vi "SLSC Convert EDS Properties and Commands to Tree Control.vi"(4 "Enum string":cluster{"name":string, "enum":string}[](array[cluster]), 6 "Item Indent":i32, 9 "commands":T1[](array[typedef]), 10 "properties":T2[](array[typedef]), 11 "Child Tag":string) -> (3 "Tree Items":T3(array[cluster]))   [LabVIEW 2017, in "SLSC Tree Control.lvlib"]
doc: "Convert the properties and commands datatypes to a Tree Control items."
uses:
  SLSC Tree Control.lvlib
  Ctrl/Property.ctl
  Ctrl/command.ctl
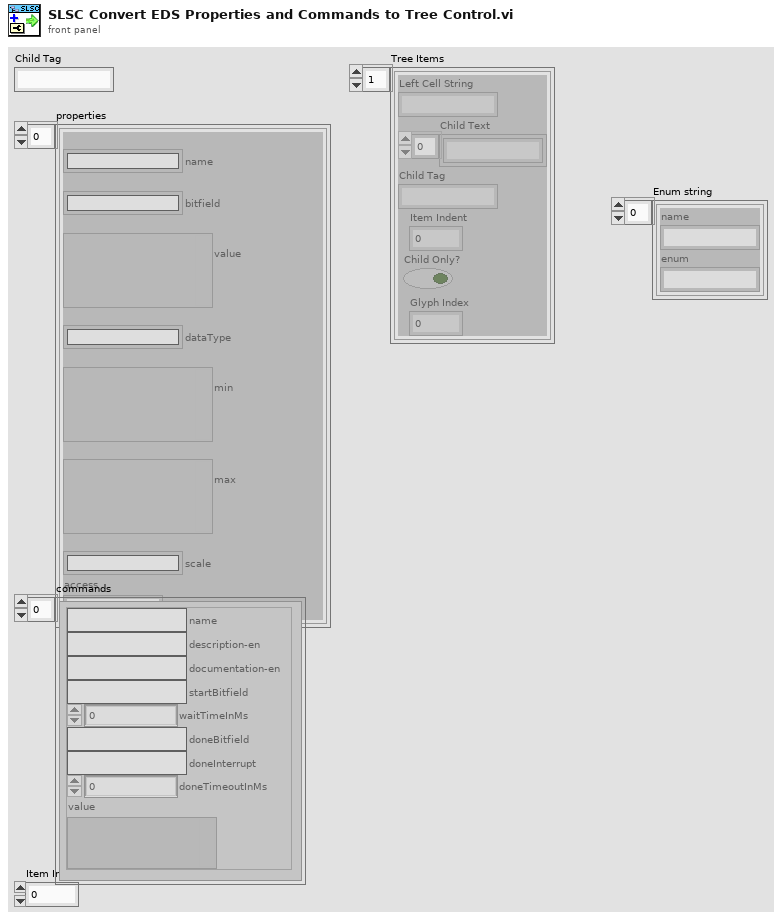
[diagram p1: front panel]
types:
  T1 = typedef "command.ctl" = cluster{"name":string, "description-en":string, "documentation-en":string, "startBitfield":string, "waitTimeInMs":i32, "doneBitfield":string, "doneInterrupt":string, "doneTimeoutInMs":i32, "value":variant}
  T2 = typedef "Property.ctl" = cluster{"name":string, "bitfield":string, "value":variant, "dataType":string, "min":variant, "max":variant, "scale":string, "access":string}
  T3 = cluster{"Left Cell String":string, "Child Text":string[], "Child Tag":string, "Item Indent":i32, "Child Only?":bool, "Glyph Index":i32}[]
  T4 = cluster{"Left Cell String":string, "Child Text":string[], "Child Tag":string, "Item Indent":i32, "Child Only?":bool, "Glyph Index":i32, "offline value":variant}
  T5 = cluster{"Left Cell String":string, "Child Text":string[], "Child Tag":string, "Item Indent":i32, "Child Only?":bool, "Glyph Index":i32, "offline value":variant}[]
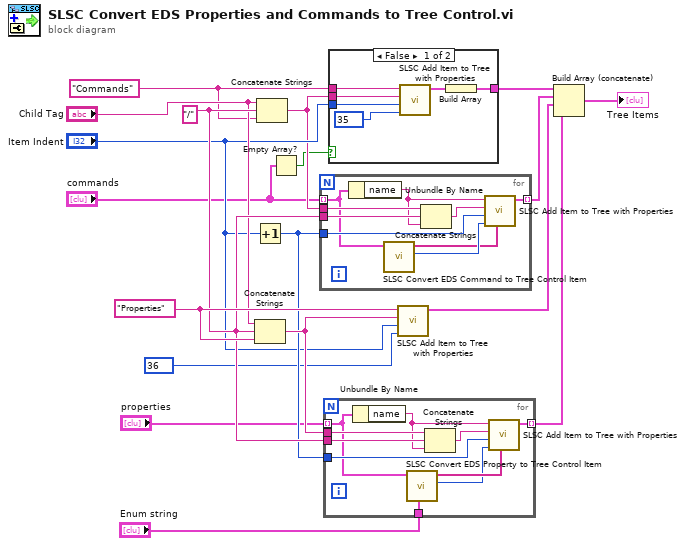
[diagram p0: block diagram]
diagram:
  w16 = "Properties" ("Left Cell String")
  w4 = "Commands" ("Left Cell String")
  w15 = "/" ("string")
  n1 = Increment(x="Item Indent") -> (x+1=w12:i32)
  n2 = Concatenate Strings("Child Tag", w15, w16) -> (w13:string)
  n3 = Concatenate Strings("Child Tag", w15, w4) -> (w7:string)
  n4 = Empty Array?(array="commands") -> (empty?=w2:bool)
  n5 = for {
    tunnel: w7 -> [w27]
    tunnel: [w25] -> w5 mode=indexing
    tunnel: "commands" -> [w21] mode=indexing
    tunnel: w12 -> [w26]
    tunnel: w15 -> [w24]
    n6 = Unbundle By Name(w21) -> ("name"=w22:string)
    n7 = call "SLSC Convert EDS Command to Tree Control Item.vi"("command"=w21) -> ("Glyph"=w20:i32, "Child Text"=w19:string[])  [unwired: 9 in]
    n8 = Concatenate Strings(w27, w24, w22) -> (w23:string)
    n9 = call "SLSC Add Item to Tree with Properties.vi"("Child Text"=w19, "Glyph Index"=w20, "Item indent"=w26, "Child Tag"=w23, "Left Cell String"=w22) -> ("Item"=w25:T4)  [unwired: 6 in]
  }
  n10 = for {
    tunnel: w13 -> [w37]
    tunnel: [w35] -> w18 mode=indexing
    tunnel: "properties" -> [w31] mode=indexing
    tunnel: w12 -> [w36]
    tunnel: w15 -> [w34]
    tunnel: "Enum string" -> [w28]
    n11 = Unbundle By Name(w31) -> ("name"=w32:string)
    n12 = call "SLSC Convert EDS Property to Tree Control Item.vi"("Enum string"=w28, "property"=w31) -> ("Glyph"=w29:i32, "Child Text"=w30:string[])  [unwired: 8 in]
    n13 = Concatenate Strings(w37, w34, w32) -> (w33:string)
    n14 = call "SLSC Add Item to Tree with Properties.vi"("Child Text"=w30, "Glyph Index"=w29, "Item indent"=w36, "Child Tag"=w33, "Left Cell String"=w32) -> ("Item"=w35:T4)  [unwired: 6 in]
  }
  n15 = case shown="False" w2 {
    tunnel: "Item Indent" -> [w43 _]
    tunnel: w7 -> [w42 _]
    tunnel: [w38 _] -> w6
    tunnel: w4 -> [w39 _]
    frame False {
      n16 = call "SLSC Add Item to Tree with Properties.vi"("Glyph Index"=35, "Item indent"=w43, "Child Tag"=w42, "Left Cell String"=w39) -> ("Item"=w41:T4)  [unwired: 7 in]
      n17 = Build Array(w41) -> (w38:T5)
    }
    frame True {
    }
  }
  n18 = call "SLSC Add Item to Tree with Properties.vi"("Glyph Index"=36, "Item indent"="Item Indent", "Child Tag"=w13, "Left Cell String"=w16) -> ("Item"=w17:T4)  [unwired: 7 in]
  n19 = Build Array (concatenate)(w6, w5, w17, w18) -> (→"Tree Items":T5)
